vi "Final_measure Y vs Voltage.vi"() -> ()   [LabVIEW 2020]
uses:
  <vilib>/DAQmx/write.llb/DAQmx Write (Analog Wfm 1Chan NSamp).vi
  <vilib>/Utility/file.llb/Write Delimited Spreadsheet (DBL).vi
  <vilib>/DAQmx/create/channels.llb/DAQmx Create Channel (AO-Voltage-Basic).vi
  <vilib>/DAQmx/configure/timing.llb/DAQmx Timing (Sample Clock).vi
  <vilib>/DAQmx/miscellaneous.llb/DAQmx Fill In Error Info.vi
  <vilib>/DAQmx/create/channels.llb/DAQmx Create Channel (CO-Pulse Generation-Frequency).vi
  <vilib>/DAQmx/configure/timing.llb/DAQmx Timing (Implicit).vi
  <resource>/objmgr/daqmx.rc
panel:
  in  "file path to save datapoints generated by labview code":path=path "C:/Users/Hannah/Downloads/Voltage postions_100.txt"
  out "x/y 2":dbl=0.0101010101010101
  in  "Number of frames":dbl=99.0
  out "Maximum Voltage value at top of FOV":dbl=0.208
  in  "Voltage value at bottom of FOV":dbl=-0.286
  out "x*y":dbl=496.0
  out "x/y":dbl=5.01010101010101
  in  "Voltage value at top of FOV":dbl=0.243
  out "x+y":dbl=496.0
  out "# Samples written per channel":u32=100
  out "actual frequency":dbl=10.0
  in  "stop":bool
  out "Signal input to voice coil (blue)":dbl[](graph)=[-0.286, -0.28065656565656566, -0.2753131313131313, -0.26996969696969697, -0.26462626262626265, -0.2592828282828283, -0.25393939393939396, -0.2485959595959596, -0.24325252525252525, -0.2379090909090909, -0.2325656565656566, -0.22722222222222224, -0.22187878787878787, -0.21653535353535353, -0.2111919191919192, -0.20584848484848484, -0.20050505050505052, -0.19516161616161617, -0.1898181818181818, -0.18447474747474746, -0.17913131313131314, -0.17378787878787877, -0.16844444444444445, -0.1631010101010101, -0.15775757575757576, -0.15241414141414142, -0.14707070707070707, -0.14172727272727273, -0.13638383838383838, -0.13104040404040404, -0.1256969696969697, -0.12035353535353537, -0.115010101010101, -0.10966666666666666, -0.10432323232323233, -0.09897979797979797, -0.09363636363636363, -0.0882929292929293, -0.08294949494949495, -0.0776060606060606, -0.07226262626262626, -0.06691919191919192, -0.06157575757575756, -0.05623232323232324, -0.050888888888888886, -0.045545454545454535, -0.04020202020202021, -0.03485858585858585, -0.0295151515151515, -0.02417171717171715, -0.01882828282828285, -0.013484848484848499, -0.008141414141414146, -0.0027979797979797924, 0.002545454545454561, 0.007888888888888914, 0.01323232323232321, 0.018575757575757565, 0.023919191919191916, 0.02926262626262627, 0.034606060606060626, 0.03994949494949498, 0.045292929292929274, 0.050636363636363625, 0.05597979797979798, 0.061323232323232335, 0.06666666666666668, 0.07201010101010098, 0.07735353535353534, 0.08269696969696969, 0.08804040404040404, 0.09338383838383839, 0.09872727272727275, 0.10407070707070705, 0.1094141414141414, 0.11475757575757575, 0.1201010101010101, 0.12544444444444447, 0.13078787878787881, 0.1361313131313131, 0.14147474747474745, 0.14681818181818182, 0.15216161616161616, 0.1575050505050505, 0.16284848484848488, 0.16819191919191917, 0.17353535353535351, 0.1788787878787879, 0.18422222222222223, 0.18956565656565658, 0.19490909090909095, 0.20025252525252524, 0.20559595959595958, 0.21093939393939393, 0.2162828282828283, 0.22162626262626264, 0.226969696969697, 0.2323131313131313, 0.2376565656565657, 0.243]
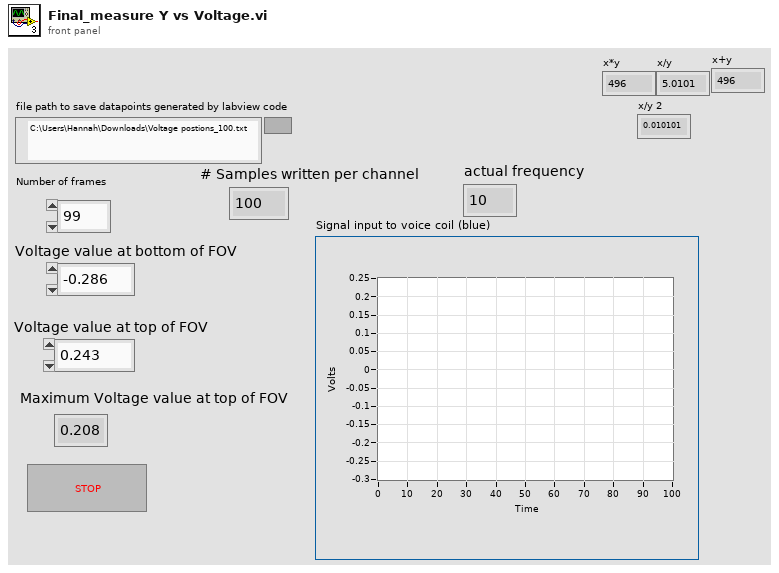
[diagram p1: front panel]
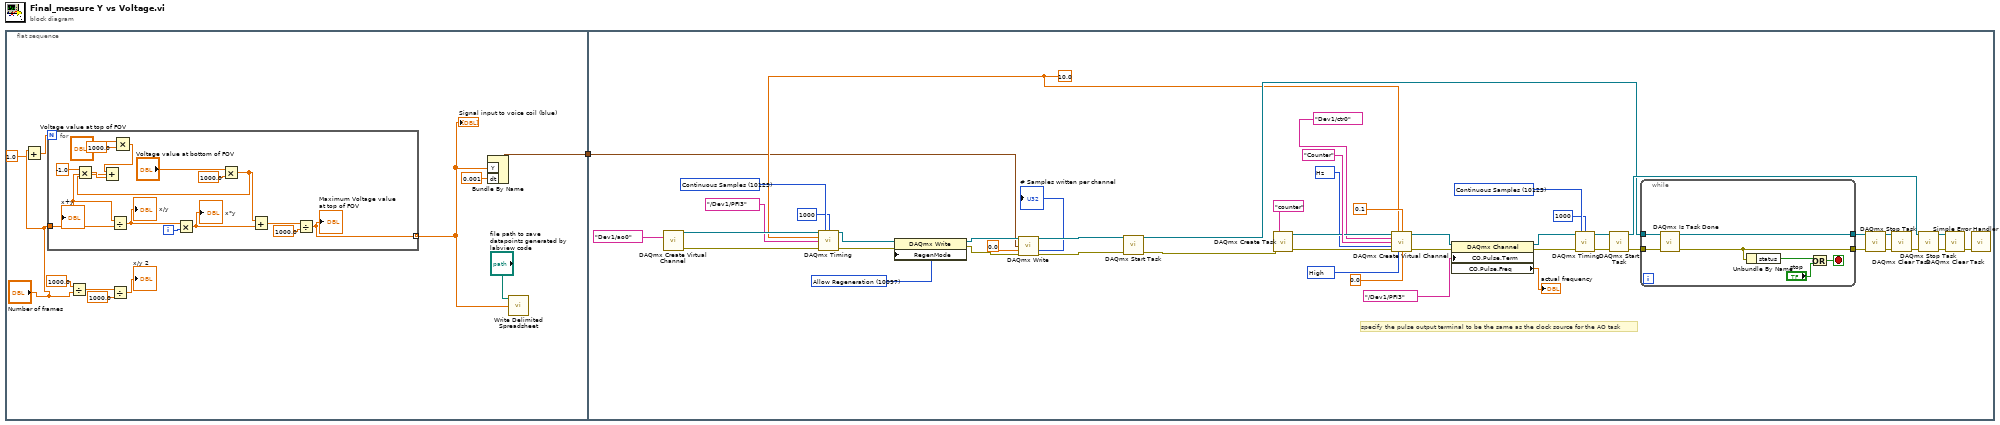
[diagram p0: block diagram]
diagram:
  n1 = flat-sequence {
    tunnel: [w4] -> w1
    tunnel: w1 -> [w29]
    frame #0 {
      n2 = Add(x="Number of frames", y=1.0) -> (x+y=w10:dbl)
      n3 = for {
        N: w10 -> [_]
        tunnel: [w20] -> w2 mode=indexing
        tunnel: "Number of frames" -> [w27]
        i -> [w28]
        n4 = Multiply(x="Voltage value at top of FOV", y=1000.0) -> (x*y=w16:dbl)
        n5 = Multiply(x="Voltage value at bottom of FOV", y=1000.0) -> (x*y=w18:dbl)
        n6 = Multiply(x=-1.0, y=w18) -> (x*y=w17:dbl)
        n7 = Add(x=w16, y=w17) -> (x+y=w13:dbl)
        "x+y" <- w13
        n8 = Divide(x=w13, y=w27) -> (x/y=w25:dbl)
        "x/y" <- w25
        n9 = Multiply(x=w25, y=w28) -> (x*y=w26:dbl)
        "x*y" <- w26
        n10 = Add(x=w18, y=w26) -> (x+y=w21:dbl)
        n11 = Divide(x=w21, y=1000.0) -> (x/y=w20:dbl)
        "Maximum Voltage value at top of FOV" <- w20
      }
      "Signal input to voice coil (blue)" <- w2
      n12 = Divide(x=1000.0, y="Number of frames") -> (x/y=w9:dbl)
      n13 = Divide(x=w9, y=1000.0) -> (x/y=→"x/y 2":dbl)
      n14 = Bundle By Name("Y"=w2, "dt"=0.001) -> (w4:waveform(dbl))  [unwired: 1 in]
      n15 = call-poly <vilib>:"Write Delimited Spreadsheet.vi"("file path (dialog if empty)"="file path to save datapoints generated by labview code", "1D data"=w2) -> ()  [unwired: 12 in, 2 out]
    }
    frame #1 {
      w33 = 10097 items=["Allow Regeneration"=10097, "Do Not Allow Regeneration"=10158] ("RegenMode")
      w42 = 10192 items=["High"=10192, "Low"=10214] ("idle state")
      w43 = 10373 items=["Hz"=10373] ("units")
      w71 = 10123 items=["Finite Samples"=10178, "Continuous Samples"=10123, "Hardware Timed Single Point"=12522] ("sample mode")
      w32 = 10.0 ("rate")
      w74 = 10123 items=["Finite Samples"=10178, "Continuous Samples"=10123, "Hardware Timed Single Point"=12522] ("sample mode")
      # "specify the pulse output terminal to be the same as the clock source for the AO task"
      n16 = call-poly <vilib>:"DAQmx Create Virtual Channel.vi"("physical channels"=tag "Dev1/ao0") -> ("task out"=w76:refnum<k21>, "error out"=w75:errorcluster)  [unwired: 13 in]
      n17 = call-poly <vilib>:"DAQmx Timing.vi"("task/channels in"=w76, "sample mode"=w74, "samples per channel"=1000, "rate"=w32, "source"=tag "/Dev1/PFI3", "error in"=w75) -> ("task out"=w37:refnum<k21>, "error out"=w36:errorcluster)  [unwired: 8 in]
      n18 = property class="DAQmx Write"(reference=w37, error in=w36, "RegenMode"=w33) -> (reference out=w35:refnum<k21>, error out=w34:errorcluster)
      n19 = call-poly <vilib>:"DAQmx Write.vi"("task/channels in"=w35, "data"=w29, "timeout"=0.0, "error in"=w34) -> ("task out"=w49:refnum<k21>, "number of samples written per channel"=→"# Samples written per channel":u32, "error out"=w48:errorcluster)  [unwired: 9 in]
      n20 = call <vilib>:"DAQmx Start Task.vi"("task/channels in"=w49, "error in"=w48) -> ("task out"=w41:refnum<k21>, "error out"=w40:errorcluster)  [unwired: 12 in]
      n21 = call <vilib>:"DAQmx Create Task.vi"("new task name"="counter", "error in"=w40) -> ("task out"=w67:refnum<k21>, "error out"=w65:errorcluster)  [unwired: 12 in]
      n22 = call-poly <vilib>:"DAQmx Create Virtual Channel.vi"("task in"=w67, "frequency"=w32, "duty cycle"=0.1, "counter"=tag "Dev1/ctr0", "name to assign"="Counter", "units"=w43, "error in"=w65, "idle state"=w42, "initial delay"=0.0) -> ("task out"=w64:refnum<k21>, "error out"=w63:errorcluster)  [unwired: 5 in]
      n23 = property class="DAQmx Channel"(reference=w64, error in=w63, "CO.Pulse.Term"=tag "/Dev1/PFI3") -> (reference out=w60:refnum<k21>, error out=w61:errorcluster, "CO.Pulse.Freq"=→"actual frequency":dbl)
      n24 = call-poly <vilib>:"DAQmx Timing.vi"("task/channels in"=w60, "sample mode"=w71, "samples per channel"=1000, "error in"=w61) -> ("task out"=w70:refnum<k21>, "error out"=w69:errorcluster)  [unwired: 10 in]
      n25 = call <vilib>:"DAQmx Start Task.vi"("task/channels in"=w70, "error in"=w69) -> ("task out"=w59:refnum<k21>, "error out"=w50:errorcluster)  [unwired: 12 in]
      n26 = while {
        tunnel: w41 -> [w83]
        tunnel: w50 -> [w82]
        tunnel: [w81] -> w55
        tunnel: [w80] -> w56
        stop <- w77 stop-if-true
        n27 = call <vilib>:"DAQmx Is Task Done.vi"("task/channels in"=w83, "error in"=w82) -> ("task out"=w81:refnum<k21>, "error out"=w80:errorcluster)  [unwired: 11 in, 1 out]
        n28 = Unbundle By Name(w80) -> ("status"=w79:bool)
        n29 = Or(x=w79, y="stop") -> (x .or. y?=w77:bool)
      }
      n30 = call <vilib>:"DAQmx Stop Task.vi"("task/channels in"=w55, "error in"=w56) -> ("task out"=w54:refnum<k21>, "error out"=w53:errorcluster)  [unwired: 12 in]
      n31 = call <vilib>:"DAQmx Clear Task.vi"("task in"=w54, "error in"=w53) -> ("error out"=w52:errorcluster)  [unwired: 13 in]
      n32 = call <vilib>:"DAQmx Stop Task.vi"("task/channels in"=w59, "error in"=w52) -> ("task out"=w57:refnum<k21>, "error out"=w58:errorcluster)  [unwired: 12 in]
      n33 = call <vilib>:"DAQmx Clear Task.vi"("task in"=w57, "error in"=w58) -> ("error out"=w51:errorcluster)  [unwired: 13 in]
      n34 = call <vilib>:"Simple Error Handler.vi"("error in (no error)"=w51) -> ()  [unwired: 4 in, 5 out]
    }
  }
